vi "PQgetTable.vi"(8 "error in":errorcluster, 10 "query":string, 11 "conn":u64) -> (0 "error out":errorcluster, 1 "Data":string[][](array[string]), 3 "conn_out":u64, 4 "PQnFields":i64, 6 "PQnTuples":i64)   [LabVIEW 2019, in "libpqutility64.lvlib"]
uses:
  libpqutility64.lvlib
  libpqlv64/src/PQgetvalue.vi
  libpqlv64/src/PQnfields.vi
  libpqlv64/src/PQntuples.vi
  libpqlv64/libpqlv64.lvlib
panel:
  out "PQsendQuery":i64
  out "PQresultStatus":T1(ring)
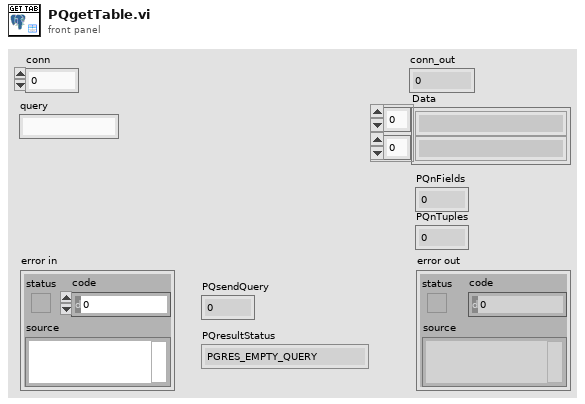
[diagram p1: front panel]
types:
  T1 = enum32{"PGRES_EMPTY_QUERY", "PGRES_COMMAND_OK", "PGRES_TUPLES_OK", "PGRES_COPY_OUT", "PGRES_COPY_IN", "PGRES_BAD_RESPONSE", "PGRES_NONFATAL_ERROR", "PGRES_FATAL_ERROR"}
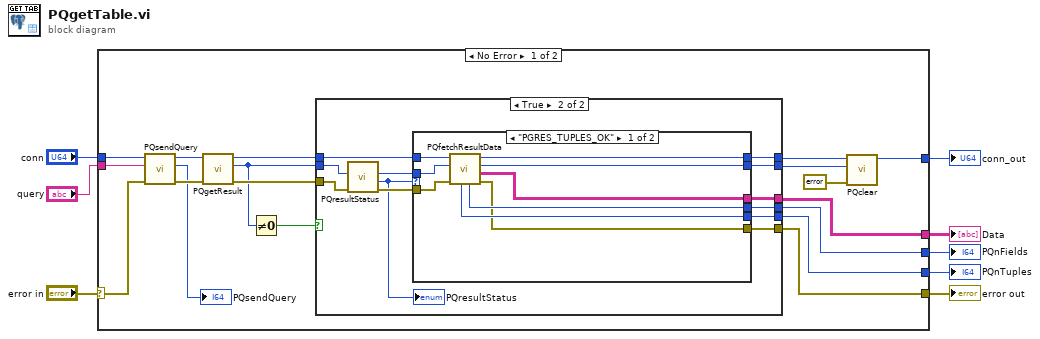
[diagram p0: block diagram]
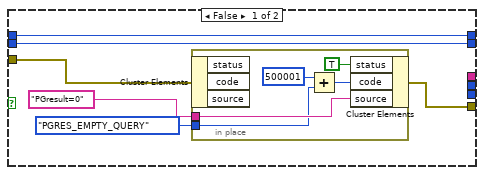
[diagram p2: hidden frame]
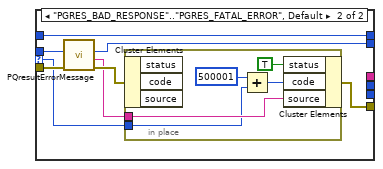
[diagram p3: hidden frame]
diagram:
  n1 = case shown="No Error" "error in" {
    selector: "error in" -> [w19 w73]
    tunnel: "conn" -> [w20 w72]
    tunnel: [w21 w73] -> w8
    tunnel: [w13 _] -> w6
    tunnel: "query" -> [w16 _]
    tunnel: [w14 _] -> w4
    tunnel: [w15 _] -> w3
    tunnel: [w9 w72] -> w1
    frame No Error {
      n2 = call "PQsendQuery.vi"("error in (no error)"=w19, "query"=w16, "conn"=w20) -> ("error out"=w26:errorcluster, "PQsendQuery"=→"PQsendQuery":i64, "conn_out"=w18:u64)  [unwired: 6 in]
      n3 = call "PQgetResult.vi"("error in (no error)"=w26, "conn"=w18) -> ("error out"=w25:errorcluster, "PGresult"=w24:u64, "conn_out"=w17:u64)  [unwired: 7 in]
      n4 = Not Equal To 0?(x=w24) -> (x != 0?=w23:bool)
      n5 = case shown="True" w23 {
        tunnel: w25 -> [w28 w49]
        tunnel: w17 -> [w31 w48]
        tunnel: [_ w46] -> w13
        tunnel: [_ w45] -> w14
        tunnel: [w27 w44] -> w21
        tunnel: w24 -> [w32 w42]
        tunnel: [_ w43] -> w15
        tunnel: [w32 w40] -> w10
        tunnel: [w31 w38] -> w11
        frame False {
          n6 = in-place {
            in-place-border: "PGresult=0" ("source") -> [w37]
            in-place-border: T1."PGRES_EMPTY_QUERY" ("PQresultStatus") -> [w34]
            n7 = in-place-cluster #1(w28) -> ()  [unwired: 3 out]
            n8 = Add(x=u32 500001, y=w34) -> (x+y=w33:u32)
            n9 = in-place-cluster #1("status"=TRUE, "code"=w33, "source"=w37) -> (w27:errorcluster)
          }
        }
        frame True {
          n10 = call "PQresultStatus.vi"("error in (no error)"=w49, "res"=w42) -> ("error out"=w47:errorcluster, "PQresultStatus"=w41:T1, "res out"=w39:u64)  [unwired: 7 in]
          "PQresultStatus" <- w41
          n11 = case shown="\"PGRES_TUPLES_OK\"" w41 {
            selector: w41 -> [_ w62]
            tunnel: w39 -> [w56 w64]
            tunnel: [w51 _] -> w45
            tunnel: w47 -> [w53 w66]
            tunnel: w48 -> [w57 w65]
            tunnel: [w54 _] -> w46
            tunnel: [w50 w59] -> w44
            tunnel: [w52 _] -> w43
            tunnel: [w55 w60] -> w40
            tunnel: [w58 w65] -> w38
            frame "PGRES_TUPLES_OK" {
              n12 = call "PQfetchResultData.vi"("error in"=w53, "res"=w56, "conn"=w57) -> ("error out"=w50:errorcluster, "Data"=w54:string[][], "res_out"=w55:u64, "conn_out"=w58:u64, "PQnFields"=w51:i64, "PQnTuples"=w52:i64)  [unwired: 3 in]
            }
            frame "PGRES_BAD_RESPONSE".."PGRES_FATAL_ERROR", Default {
              n13 = call "PQresultErrorMessage.vi"("error in (no error)"=w66, "res"=w64) -> ("error out"=w63:errorcluster, "PQresultErrorMessage"=w61:string, "res out"=w60:u64)  [unwired: 7 in]
              n14 = in-place {
                in-place-border: w61 -> [w71]
                in-place-border: w62 -> [w68]
                n15 = in-place-cluster #2(w63) -> ()  [unwired: 3 out]
                n16 = Add(x=u32 500001, y=w68) -> (x+y=w67:u32)
                n17 = in-place-cluster #2("status"=TRUE, "code"=w67, "source"=w71) -> (w59:errorcluster)
              }
            }
          }
        }
      }
      n18 = call "PQclear.vi"("error in"=errorcluster {"status"=FALSE, "code"=0, "source"=""} ("error in (no error)"), "res"=w10, "conn"=w11) -> ("conn_out"=w9:u64)  [unwired: 7 in, 1 out]
    }
    frame Error {
    }
  }
  "conn_out" <- w1
  "error out" <- w8
  "Data" <- w6
  "PQnFields" <- w4
  "PQnTuples" <- w3
